vi "usrp get rx subdev name.vi"(7 "strbuffer_len":u64, 8 "error in (no error)":errorcluster, 9 "rx_subdev_name_out":string, 10 "chan":u64, 11 "h":u64) -> (0 "error out":errorcluster, 1 "rx_subdev_name_out out":string, 3 "function return":u32(ring))   [LabVIEW 2023, in "uhd.lvlib"]
doc: "UHD_API uhd_error uhd_usrp_get_rx_subdev_name(\n uhd_usrp_handle h, size_t chan, char* rx_subdev_name_out, size_t strbuffer_len);"
uses:
  <userlib>/uhd/uhd.lvlib
  <userlib>/uhd/uhd.dll
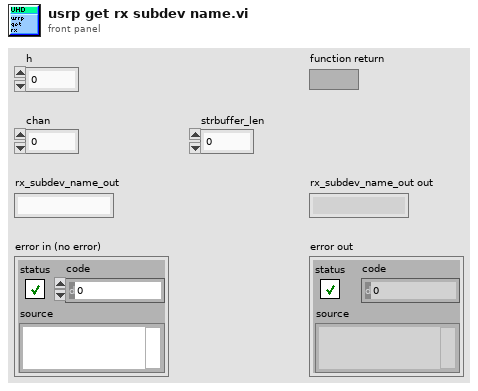
[diagram p1: front panel]
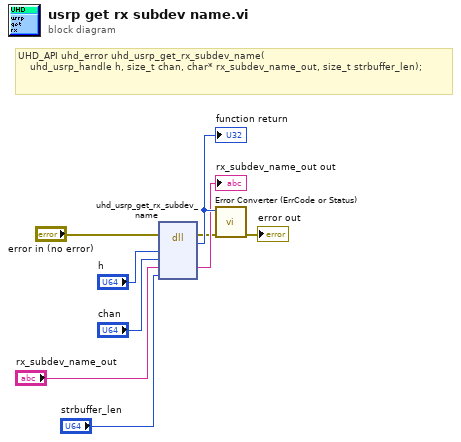
[diagram p0: block diagram]
diagram:
  # "UHD_API uhd_error uhd_usrp_get_rx_subdev_name(\n    uhd_usrp_handle h, size_t chan, char* rx_subdev_name_out, size_t strbuffer_len);"
  n1 = dll-call lib="C:/Program Files/National Instruments/LabVIEW 2023/user.lib/uhd/uhd.*" fn="uhd_usrp_get_rx_subdev_name"(error in="error in (no error)", "h"="h", "chan"="chan", "rx_subdev_name_out"="rx_subdev_name_out", "strbuffer_len"="strbuffer_len") -> (error out=w2:errorcluster, w9:u32, "rx_subdev_name_out"=→"rx_subdev_name_out out":string)  [unwired: 5 in, 1 out]
  "function return" <- w9
  n2 = call <userlib>:"Error Converter (ErrCode or Status).vi"("error in (no error)"=w2, "error code"=w9) -> ("error out"=→"error out":errorcluster)  [unwired: 9 in]
